vi "Write Photon Counter Enqueuer.vi"(10 "Actor Framework:Message Enqueuer":refnum<class "Message Enqueuer.lvclass">, 11 "Abstract Controller in":refnum<class "Abstract Controller.lvclass">) -> (3 "Abstract Controller out":refnum<class "Abstract Controller.lvclass">)   [LabVIEW 2016]
uses:
  Abstract Controller.lvclass
  C:/Program Files (x86)/National Instruments/LabVIEW 2016/vi.lib/ActorFramework/Actor/Actor.lvclass
  <vilib>/ActorFramework/Message Enqueuer/Message Enqueuer.lvclass
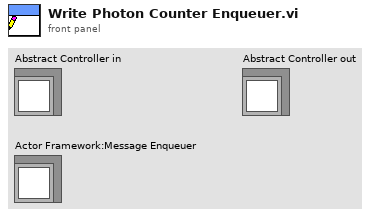
[diagram p1: front panel]
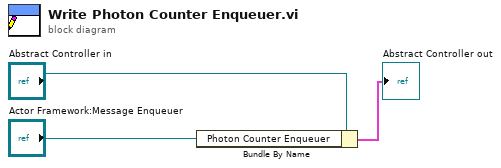
[diagram p0: block diagram]
diagram:
  n1 = Bundle By Name(cluster="Abstract Controller in", "Photon Counter Enqueuer"="Actor Framework:Message Enqueuer") -> (→"Abstract Controller out":cluster{})
